vi "GenerateGUID.vi"(11 "Keys":variant) -> (2 "GUID Cluster":cluster{u32, u16, u16, u64}, 3 "GUID String":string)   [LabVIEW 2015, in "StepNode.lvclass"]
uses:
  StepNode.lvclass
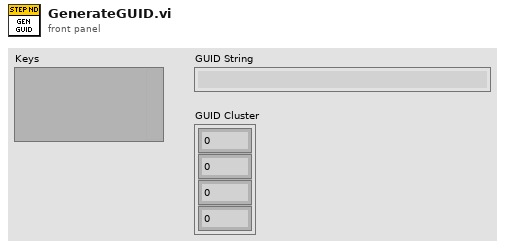
[diagram p1: front panel]
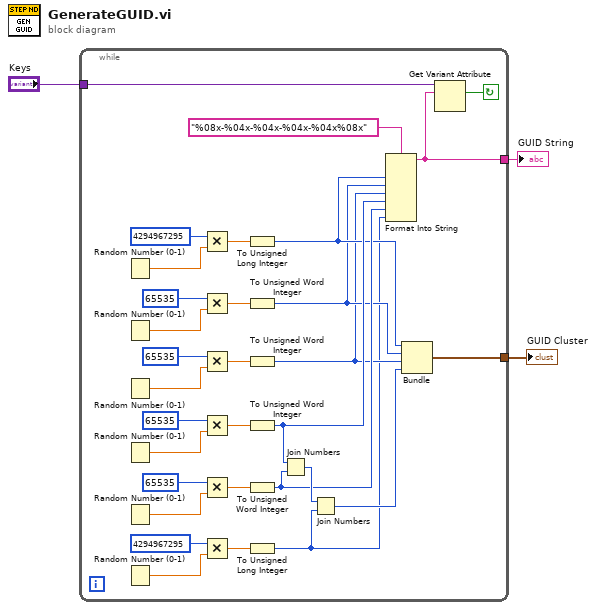
[diagram p0: block diagram]
diagram:
  n1 = while {
    tunnel: "Keys" -> [w8]
    tunnel: [w6] -> w3
    tunnel: [w5] -> w2
    stop <- w7 continue-if-true
    n2 = Random Number (0-1)() -> (number: 0 to 1=w34:dbl)
    n3 = Random Number (0-1)() -> (number: 0 to 1=w31:dbl)
    n4 = Random Number (0-1)() -> (number: 0 to 1=w30:dbl)
    n5 = Random Number (0-1)() -> (number: 0 to 1=w27:dbl)
    n6 = Random Number (0-1)() -> (number: 0 to 1=w20:dbl)
    n7 = Random Number (0-1)() -> (number: 0 to 1=w26:dbl)
    n8 = Multiply(x=u32 4294967295, y=w34) -> (x*y=w24:dbl)
    n9 = Multiply(x=u16 65535, y=w31) -> (x*y=w21:dbl)
    n10 = Multiply(x=u16 65535, y=w30) -> (x*y=w22:dbl)
    n11 = Multiply(x=u16 65535, y=w27) -> (x*y=w17:dbl)
    n12 = Multiply(x=u16 65535, y=w20) -> (x*y=w18:dbl)
    n13 = Multiply(x=u32 4294967295, y=w26) -> (x*y=w23:dbl)
    n14 = To Unsigned Long Integer(number=w24) -> (unsigned 32bit integer=w12:u32)
    n15 = To Unsigned Word Integer(number=w21) -> (unsigned 16bit integer=w11:u16)
    n16 = To Unsigned Word Integer(number=w22) -> (unsigned 16bit integer=w10:u16)
    n17 = To Unsigned Word Integer(number=w17) -> (unsigned 16bit integer=w14:u16)
    n18 = To Unsigned Word Integer(number=w18) -> (unsigned 16bit integer=w13:u16)
    n19 = To Unsigned Long Integer(number=w23) -> (unsigned 32bit integer=w4:u32)
    n20 = Join Numbers(hi=w14, lo=w13) -> ((hi.lo)=w16:u32)
    n21 = Join Numbers(hi=w16, lo=w4) -> ((hi.lo)=w9:u64)
    n22 = Format Into String(format string="%08x-%04x-%04x-%04x-%04x%08x", w12, w11, w10, w14, w13, w4) -> (resulting string=w6:string)  [unwired: 2 in, 1 out]
    n23 = Bundle(w12, w11, w10, w9) -> (w5:cluster{u32, u16, u16, u64})  [unwired: 1 in]
    n24 = Get Variant Attribute(Variant=w8, name=w6) -> (found=w7:bool)  [unwired: 2 in, 3 out]
  }
  "GUID String" <- w3
  "GUID Cluster" <- w2
